vi "poly_sub_filter_multi_wav.vi"(6 "add info? (T)":bool=TRUE, 8 "error in (no error)":errorcluster, 9 "f":i32=50 caption="base frequency (50Hz)", 10 "N":i32=3 caption="N of harmonics to remove (3)", 11 "waveforms in":waveform(dbl)[](array[waveform])) -> (0 "error out":errorcluster, 3 "waveforms out":waveform(dbl)[](array[waveform]))   [LabVIEW 2015]
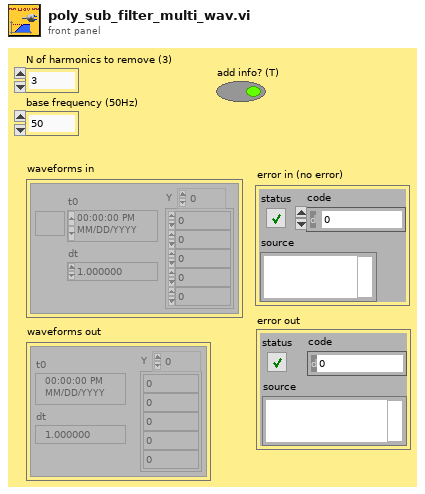
[diagram p1: front panel]
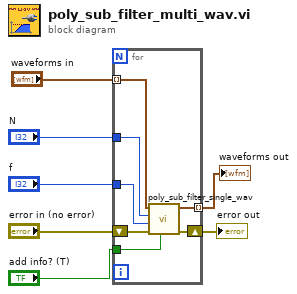
[diagram p0: block diagram]
diagram:
  n1 = for {
    tunnel: "waveforms in" -> [w14] mode=indexing
    tunnel: [w13] -> w6 mode=indexing
    shift-right: [w11] -> w4
    shift-left: "error in (no error)" -> [w12]
    tunnel: "N" -> [w10]
    tunnel: "f" -> [w9]
    tunnel: "add info? (T)" -> [w8]
    n2 = call "poly_sub_filter_single_wav.vi"("add info? (T)"=w8, "error in (no error)"=w12, "f"=w9, "N"=w10, "waveform in"=w14) -> ("error out"=w11:errorcluster, "waveform out"=w13:waveform(dbl))  [unwired: 5 in]
  }
  "error out" <- w4
  "waveforms out" <- w6
